vi "DLLPathFromAPPDir.vi"() -> (0 "error out":errorcluster, 3 "DLLPath":path)   [LabVIEW 2019]
doc: "Attemps to load pdlm_lib.dll DLL from subfolder of application path"
uses:
  <vilib>/Utility/error.llb/Error Cluster From Error Code.vi
  <vilib>/ErrorRing/Error Ring.xnode
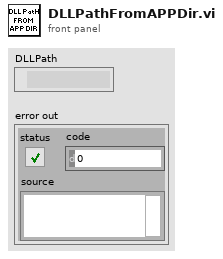
[diagram p1: front panel]
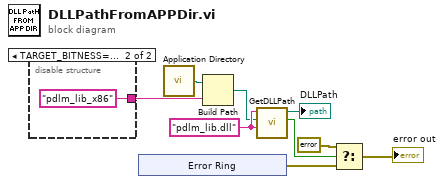
[diagram p0: block diagram]
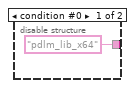
[diagram p2: hidden frame]
diagram:
  w3 = "pdlm_lib.dll" ("DllName_64bit")
  n1 = disable-structure shown="TARGET_BITNESS==32" {
    disable-tunnel: ["pdlm_lib_x64" "pdlm_lib_x86"] -> w4
    frame condition #0 {
    }
    frame condition #1 (active) {
    }
  }
  n2 = xnode "Error Ring"() -> ("sortie d'erreur"=w8:errorcluster)
  n3 = call <vilib>:"Application Directory.vi"() -> ("Application Directory"=w2:path)
  n4 = Build Path(base path=w2, name or relative path=w4) -> (appended path=w1:path)
  n5 = call <userlib>:"GetDLLPath.vi"("DllName_32bit"=w3, "PathToDLL"=w1, "DllName_64bit"=w3) -> ("file exists?"=w7:bool, "DLLPath"=→"DLLPath":path)  [unwired: 6 in, 1 out]
  n6 = Select(t=errorcluster {"status"=FALSE, "code"=0, "source"=""} ("error in (no error)"), s=w7, f=w8) -> (s? t:f=→"error out":errorcluster)
